vi "ReadNavX.vi"(1 "Terms":i32) -> ()   [LabVIEW 2017]
uses:
  <vilib>/Rock Robotics/WPI/ThirdParty/Sensors/navX/_TypeDefs/FRIC_navX_DeviceNumbersTypeDef.ctl
  Robot Global Data.vi
panel:
  out "Velocity":dbl(graph)
  out "Yaw":dbl(graph)
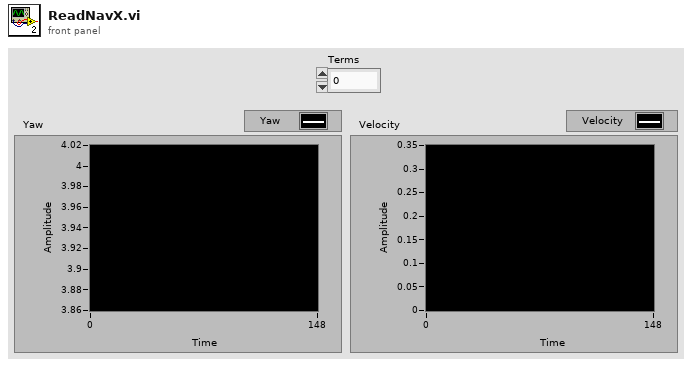
[diagram p1: front panel]
types:
  T1 = typedef "FRIC_navX_DeviceNumbersTypeDef.ctl" = enum16{"Dev0", "Dev1", "Dev2", "Dev3"}
  T2 = cluster{"Rollover":dbl, "Yaw":dbl, "Cont Yaw":dbl}
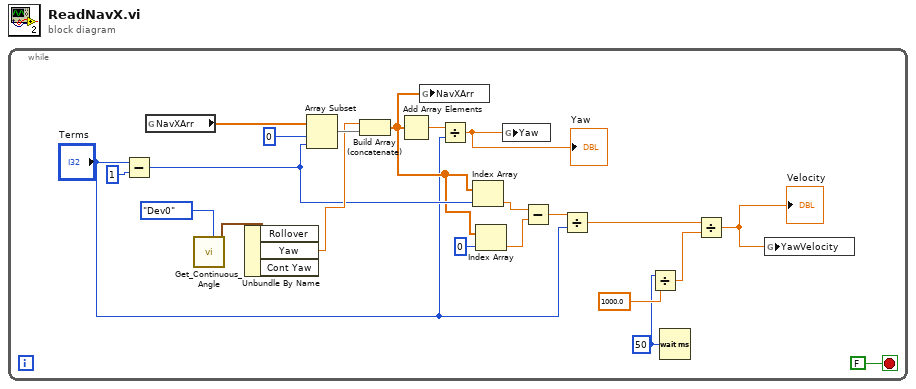
[diagram p0: block diagram]
diagram:
  n1 = while {
    stop <- FALSE stop-if-true
    w1 = u32 50 ("milliseconds to wait")
    n2 = Subtract(x="Terms", y=1) -> (x-y=w13:i32)
    n3 = global read "Robot Global Data.vi" "NavXArr"() -> (w22:dbl[])
    n4 = call <vilib>:"Get_Continuous_Angle.vi"("Device Number"=FRIC_navX_DeviceNumbersTypeDef."Dev0") -> ("Continuous Angle"=w17:T2)  [unwired: 10 in]
    n5 = Unbundle By Name(w17) -> ("Yaw"=w15:dbl)  [unwired: 2 out]
    n6 = Array Subset(array=w22, index=0, length=w13) -> (w20:dbl[])
    n7 = Build Array (concatenate)(w15, w20) -> (w11:dbl[])
    n8 = Add Array Elements(numeric array=w11) -> (sum=w18:dbl)
    n9 = global write "Robot Global Data.vi" "NavXArr"(w11) -> ()
    n10 = Divide(x=w18, y="Terms") -> (x/y=w14:dbl)
    "Yaw" <- w14
    n11 = Index Array(array=w11, index=w13) -> (element=w10:dbl)
    n12 = Index Array(array=w11, index=0) -> (element=w9:dbl)
    n13 = global write "Robot Global Data.vi" "Yaw"(w14) -> ()
    n14 = Subtract(x=w10, y=w9) -> (x-y=w8:dbl)
    n15 = Divide(x=w8, y="Terms") -> (x/y=w4:dbl)
    n16 = Divide(x=w1, y=1000.0) -> (x/y=w5:dbl)
    n17 = Wait (ms)(milliseconds to wait=w1) -> ()  [unwired: 1 out]
    n18 = Divide(x=w4, y=w5) -> (x/y=w3:dbl)
    "Velocity" <- w3
    n19 = global write "Robot Global Data.vi" "YawVelocity"(w3) -> ()
  }
